vi "Get Laser Drive.vi"(8 "error in (no error)":errorcluster, 9 "Path":path, 10 "Section":string, 11 "abstract laser driver factory in":refnum<class "abstract laser driver factory.lvclass">) -> (0 "error out":errorcluster, 2 "Laser Driver.lvclass":refnum<class "Laser Driver.lvclass">)   [LabVIEW 2022 SP3, in "abstract laser driver factory.lvclass"]
uses:
  abstract laser driver factory.lvclass
  Laser Driver/Laser Driver.lvclass
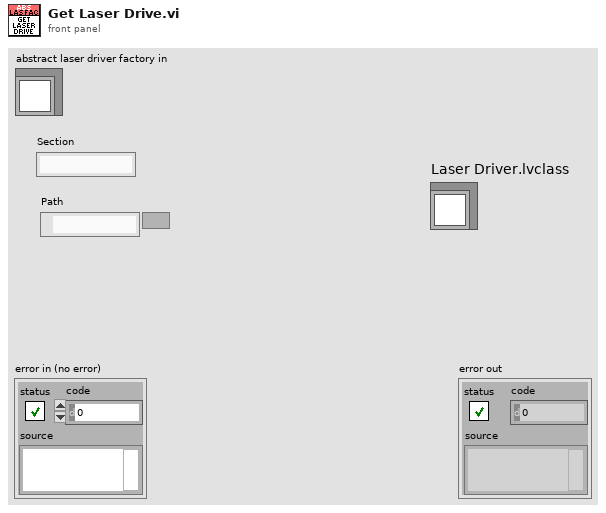
[diagram p1: front panel]
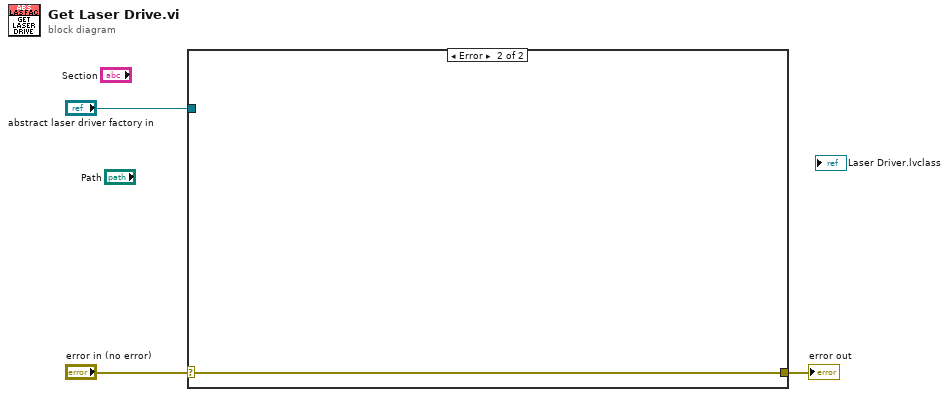
[diagram p0: block diagram]
diagram:
  n1 = case shown="Error" "error in (no error)" {
    selector: "error in (no error)" -> [w4 w5]
    tunnel: [w4 w5] -> w2
    tunnel: "abstract laser driver factory in" -> [_ _]
    frame No Error {
      # "Wire the error cluster across even in the \"No Error\"\ncase so that warnings get propagated."
    }
    frame Error {
    }
  }
  "error out" <- w2
